vi "Read Panel.vi"(8 "error in (no error)":errorcluster, 11 "Form Configuration in":refnum<class "Form Configuration.lvclass">) -> (0 "error out":errorcluster, 2 "Panel.lvlib:Panel.lvclass":refnum<class "Panel.lvclass">, 3 "Form Configuration out":refnum<class "Form Configuration.lvclass">)   [LabVIEW 2020, in "Form Configuration.lvlib" / "Form Configuration.lvclass"]
uses:
  Form Configuration.lvclass
  <vilib>/MGI/Panel Manager/Panel/Panel/Panel.lvclass
  Form Configuration.lvclass/Form Configuration.ctl
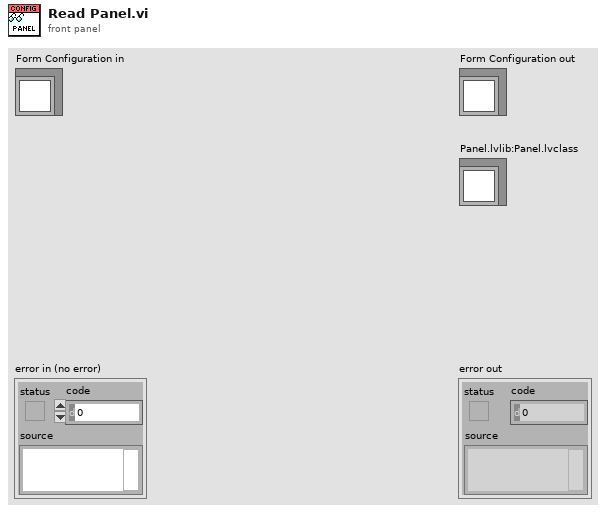
[diagram p1: front panel]
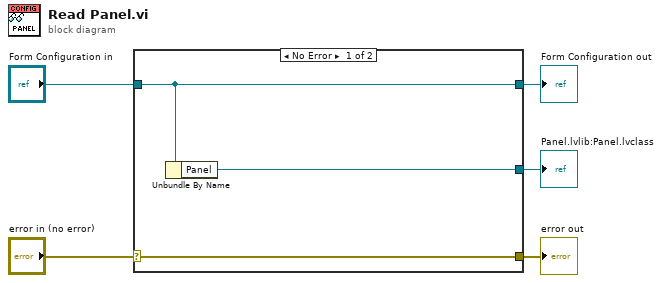
[diagram p0: block diagram]
diagram:
  n1 = case shown="No Error" "error in (no error)" {
    selector: "error in (no error)" -> [w8 w9]
    tunnel: [w8 w9] -> w4
    tunnel: [w7 w10] -> w2
    tunnel: "Form Configuration in" -> [w7 w10]
    tunnel: [w6 _] -> w1
    frame No Error {
      n2 = Unbundle By Name(w7) -> ("Panel"=w6:refnum<class "Panel.lvclass">)
    }
    frame Error {
    }
  }
  "error out" <- w4
  "Form Configuration out" <- w2
  "Panel.lvlib:Panel.lvclass" <- w1
